vi "Destroy Object.vi"(7 "Undo Text":string="Disaster", 8 "error in (no error)":errorcluster, 9 "Object Ref":refnum<vi>, 10 "BD Ref":refnum<vi>, 11 "VI Ref":refnum<vi>) -> (0 "error out":errorcluster)   [LabVIEW 2019]
doc: "Destroys the given object by deleting it, then placing fire / rubble in its location. Also sets an undo transaction so the delete can be undone."
uses:
  _Assets/Asset Enum.ctl
  <vilib>/numeric/Random Number (Range) U64.vi
  <vilib>/numeric/sub_Random U32.vi
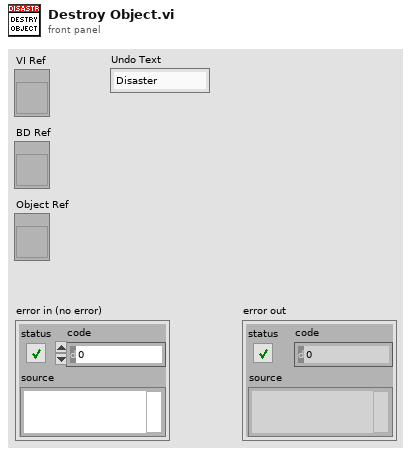
[diagram p1: front panel]
types:
  T1 = typedef "Asset Enum.ctl" = enum16{"Fire 1", "Fire 2", "Rubble"}
  T2 = typedef "LVPositionTypeDef.ctl" = cluster{"Left":i32, "Top":i32}
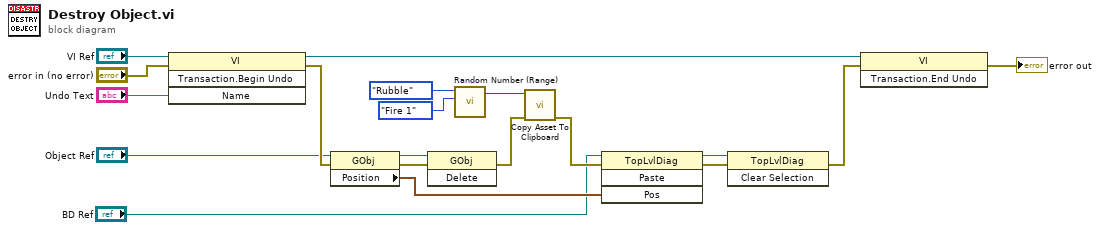
[diagram p0: block diagram]
diagram:
  n1 = invoke class="VI" method="Transaction.Begin Undo"(reference="VI Ref", error in="error in (no error)", "Name"="Undo Text") -> (reference out=w8:refnum<vi>, error out=w9:errorcluster)  [unwired: 1 in, 2 out]
  n2 = property class="GObj"(reference="Object Ref", error in=w9) -> (reference out=w19:refnum<vi>, error out=w18:errorcluster, "Position"=w17:T2)
  n3 = invoke class="GObj" method="Delete"(reference=w19, error in=w18) -> (error out=w13:errorcluster)  [unwired: 1 in, 2 out]
  n4 = call-poly <vilib>:"Random Number (Range).vi"("lower bound (0)"=Asset_Enum."Fire 1" ("Asset"), "upper bound (100)"=Asset_Enum."Rubble" ("Asset")) -> ("number"=w12:u64)  [unwired: 9 in]
  n5 = call "Copy Asset To Clipboard.vi"("error in (no error)"=w13, "Asset"=w12) -> ("error out"=w16:errorcluster)  [unwired: 9 in]
  n6 = invoke class="TopLvlDiag" method="Paste"(reference="BD Ref", error in=w16, "Pos"=w17) -> (reference out=w11:refnum<vi>, error out=w4:errorcluster)  [unwired: 1 in, 2 out]
  n7 = invoke class="TopLvlDiag" method="Clear Selection"(reference=w11, error in=w4) -> (error out=w7:errorcluster)  [unwired: 1 in, 2 out]
  n8 = invoke class="VI" method="Transaction.End Undo"(reference=w8, error in=w7) -> (error out=→"error out":errorcluster)  [unwired: 1 in, 2 out]
